vi "SetResol.vi"(2 "DeviceIndex":i32, 4 "Binning":i32 min=0 max=5 step=1) -> (0 "Resolution":dbl format="%.2f", 1 "Error":bool)   [LabVIEW 2011]
uses:
  MT Scan/SubVIs/hhlib.dll
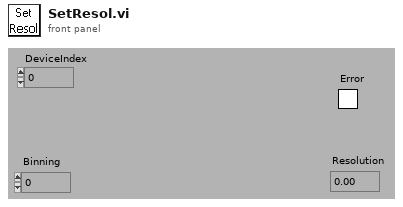
[diagram p1: front panel]
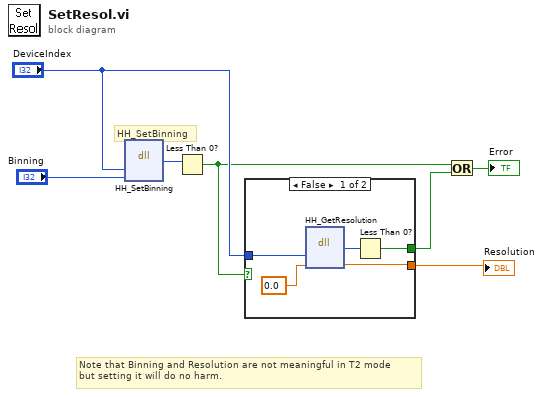
[diagram p0: block diagram]
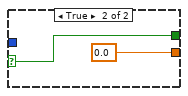
[diagram p2: hidden frame]
diagram:
  # "HH_SetBinning"
  # "Note that Binning and Resolution are not meaningful in T2 mode\nbut setting it will do no harm."
  n1 = dll-call lib="C:/Users/Core-FCS/Desktop/AbelFCS/MT Scan/SubVIs/hhlib.dll" fn="HH_SetBinning"("devidx"="DeviceIndex", "Range"="Binning") -> (w7:i32)  [unwired: 5 in, 2 out]
  n2 = Less Than 0?(x=w7) -> (x < 0?=w2:bool)
  n3 = case shown="False" w2 {
    selector: w2 -> [_ w13]
    tunnel: [w10 0.0] -> w4
    tunnel: "DeviceIndex" -> [w12 _]
    tunnel: [w8 w13] -> w3
    frame False {
      n4 = dll-call lib="C:/Users/Core-FCS/Desktop/AbelFCS/MT Scan/SubVIs/hhlib.dll" fn="HH_GetResolution"("devidx"=w12, "resolution"=0.0) -> (w9:i32, "resolution"=w10:dbl)  [unwired: 4 in, 2 out]
      n5 = Less Than 0?(x=w9) -> (x < 0?=w8:bool)
    }
    frame True {
    }
  }
  "Resolution" <- w4
  n6 = Or(x=w2, y=w3) -> (x .or. y?=→"Error":bool)
